vi "表换线提示.vi"(8 "error in (no error)":errorcluster caption="错误输入（无错误）", 11 "34401A 输入":refnum<class "34401A.lvclass">) -> (0 "error out":errorcluster caption="错误输出", 3 "34401A 输出":refnum<class "34401A.lvclass">)   [LabVIEW 2020, in "34401A.lvlib" / "34401A.lvclass"]
uses:
  34401A.lvclass
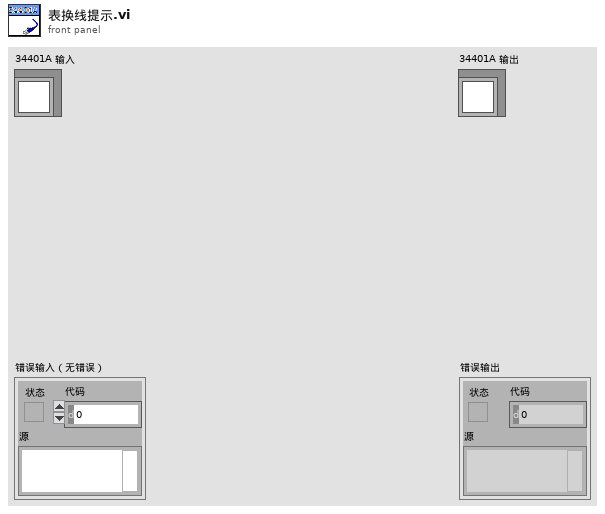
[diagram p1: front panel]
types:
  T1 = enum16{"DC Voltage", "AC Voltage", "Resistance", "DC Current", "AC Current"}
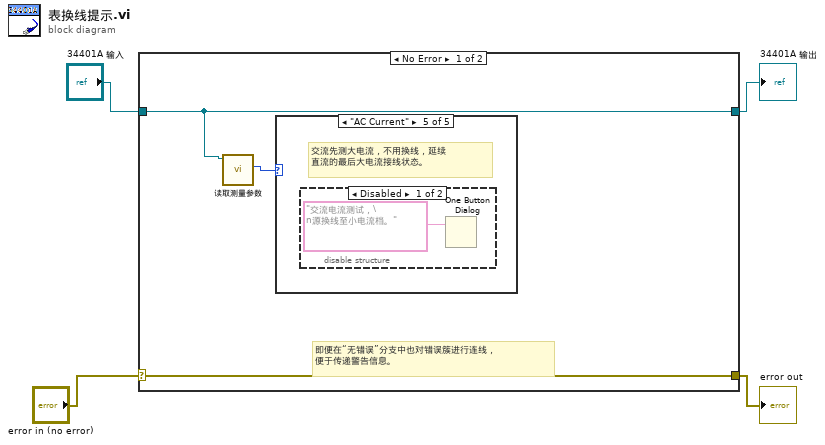
[diagram p0: block diagram]
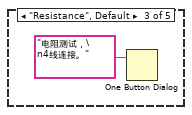
[diagram p4: hidden frame]
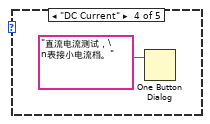
[diagram p5: hidden frame]
diagram:
  n1 = case shown="No Error" "error in (no error)" {
    selector: "error in (no error)" -> [w7 w12]
    tunnel: [w7 w12] -> w2
    tunnel: [w6 w11] -> w3
    tunnel: "34401A 输入" -> [w6 w11]
    frame No Error {
      # "即便在“无错误”分支中也对错误簇进行连线，\n便于传递警告信息。"
      n2 = call "读取测量参数.vi"("数字多用表接口输入"=w6) -> ("测量参数"=w5:T1)  [unwired: 8 in, 2 out]
      n3 = case shown="\"AC Current\"" w5 {
        frame "DC Voltage" {
        }
        frame "AC Voltage" {
        }
        frame "Resistance", Default {
          n4 = One Button Dialog(message="电阻测试，\n4线连接。") -> ()  [unwired: 1 in, 1 out]
        }
        frame "DC Current" {
          n5 = One Button Dialog(message="直流电流测试，\n表接小电流档。") -> ()  [unwired: 1 in, 1 out]
        }
        frame "AC Current" {
          # "交流先测大电流，不用换线，延续\n直流的最后大电流接线状态。"
          n6 = disable-structure shown="Disabled" {
            frame Disabled {
              n7 = One Button Dialog(message="交流电流测试，\n源换线至小电流档。") -> ()  [unwired: 1 in, 1 out]
            }
            frame Enabled {
            }
          }
        }
      }
    }
    frame Error {
    }
  }
  "error out" <- w2
  "34401A 输出" <- w3
